vi "Test Oscilloscope.vi"() -> ()   [LabVIEW 2020]
uses:
  Osciloscope Tektronix.lvlib
panel:
  out "Waveform Graph":waveform(dbl)(graph)
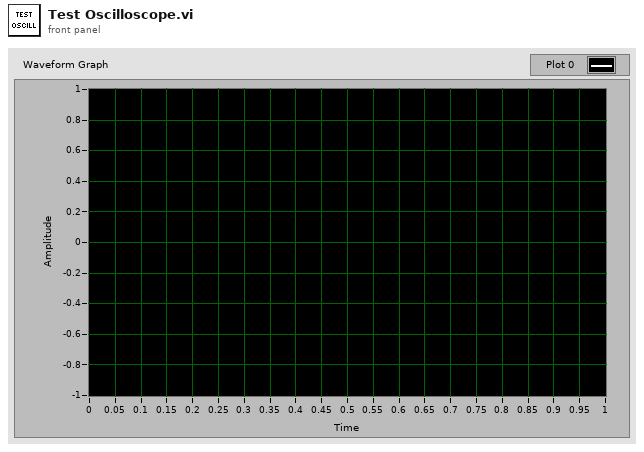
[diagram p1: front panel]
types:
  T1 = cluster{"Source (0: Channel 1)":u16, "Timeout (10000 ms)":u32}
  T2 = typedef "Osciloscope Tektronix.lvlib/Broadcast Events--cluster.ctl" = cluster{"Module Did Init":refnum<user-event>, "Status Updated":refnum<user-event>, "Error Reported":refnum<user-event>, "Module Did Stop":refnum<user-event>, "Update Module Execution Status":refnum<user-event>, "Oscilloscopes List":refnum<user-event>}
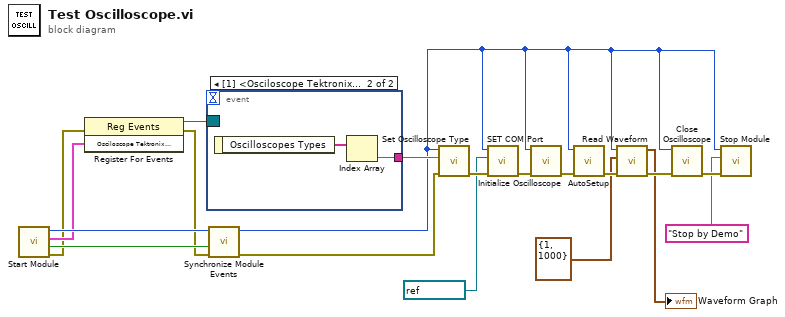
[diagram p0: block diagram]
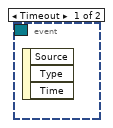
[diagram p2: hidden frame]
diagram:
  n1 = call "Start Module.vi"() -> ("error out"=w15:errorcluster, "Wait for Event Sync?"=w18:bool, "Osciloscope Tektronix Broadcast Events"=w16:T2, "Module ID"=w19:i32)  [unwired: 8 in]
  n2 = register-events(error in=w15, w16) -> (reference out=w17:refnum<event-registration>, error out=w14:errorcluster)  [unwired: 1 in]
  n3 = event shown="[1] <Osciloscope Tektronix Broadcast Events.Oscilloscopes List>: User Event" {
    selector: w17 -> [_ _]
    dyn-events: _ -> [_ _]
    timeout: _ -> [_ _]
    tunnel: [_ w20] -> w12
    event Timeout {
      n4 = event-data() -> ()  [unwired: 1 in, 3 out]
    }
    event User Event {
      n5 = event-data() -> ("Oscilloscopes Types"=w21:string[])  [unwired: 1 in]
      n6 = Index Array(array=w21) -> (element=w20:string)  [unwired: 1 in]
    }
  }
  n7 = call "Synchronize Module Events.vi"("error in"=w14, "Wait for Event Sync?"=w18, "Module ID in"=w19) -> ("error out"=w13:errorcluster, "Module ID out"=w3:i32)  [unwired: 7 in]
  n8 = call "Set Oscilloscope Type.vi"("error in"=w13, "Oscilloscope"=w12, "Module ID"=w3) -> ("error out"=w11:errorcluster)  [unwired: 8 in]
  n9 = call "SET COM Port.vi"("error in"=w11, "COM"=refnum<visa-resource-name> "COM1", "Module ID"=w3) -> ("error out"=w9:errorcluster)  [unwired: 8 in]
  n10 = call "Initialize Oscilloscope.vi"("error in"=w9, "Module ID"=w3) -> ("error out"=w6:errorcluster)  [unwired: 9 in]
  n11 = call "AutoSetup.vi"("error in"=w6, "Module ID"=w3) -> ("error out"=w8:errorcluster)  [unwired: 9 in]
  n12 = call "Read Waveform.vi"("error in"=w8, "Parameters 3"=T1 {"Source (0: Channel 1)"=1, "Timeout (10000 ms)"=1000}, "Module ID"=w3) -> ("error out"=w7:errorcluster, "Waveform Graph"=→"Waveform Graph":waveform(dbl))  [unwired: 6 in, 1 out]
  n13 = call "Close Oscilloscope.vi"("error in"=w7, "Module ID"=w3) -> ("error out"=w4:errorcluster)  [unwired: 9 in]
  n14 = call "Stop Module.vi"("error in (no error)"=w4, "Origin"="Stop by Demo", "Module ID"=w3) -> ()  [unwired: 8 in, 1 out]
